vi "lab 9.vi"() -> ()   [LabVIEW 2021]
uses:
  <vilib>/MakerHub/LINX/Public/Peripherals/Analog/Analog Read 1 Chan.vi
  <vilib>/MakerHub/LINX/Public/Peripherals/Analog/Analog Read N Chans.vi
  <vilib>/MakerHub/LINX/Private/Local IO/LinxAnalogRead.vi
  <vilib>/MakerHub/LINX/Public/Utilities/Check Channel.vi
  <vilib>/MakerHub/LINX/Public/Utilities/Open Serial.vi
  <vilib>/MakerHub/LINX/Public/Sensors/Motion/Servo/Servo Set Pulse Width One Channel.vi
  <vilib>/MakerHub/LINX/Private/Utilties/Generate Error.vi
  <vilib>/MakerHub/LINX/LMH-LINX.lvlib
  <vilib>/MakerHub/LINX/Public/Sensors/Motion/Servo/Servo.lvlib
panel:
  in  "stop Button":bool
  in  "Servo Channel":u8
  in  "Analog Channel":u8
  out "Waveform Chart 2":dbl(graph)
  out "Waveform Chart":dbl(graph)
  in  "Serial Port":refnum<visa-resource-name>="N/A"
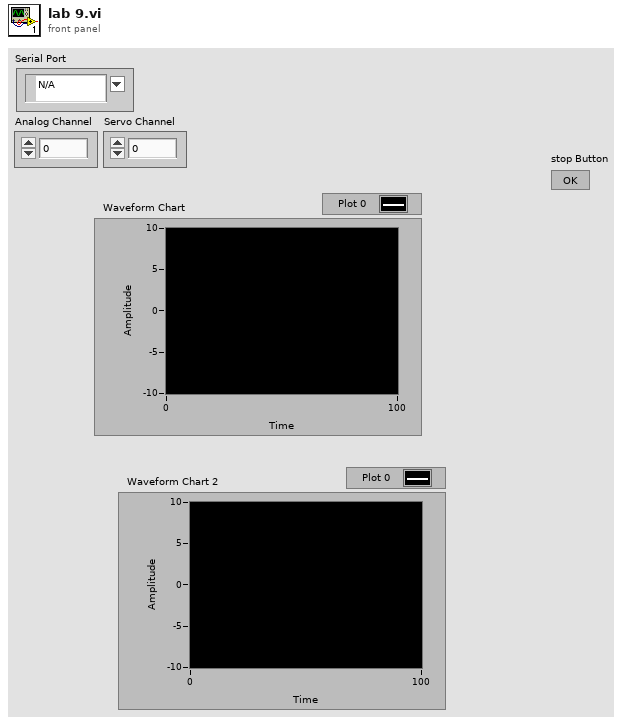
[diagram p1: front panel]
types:
  T1 = typedef "LMH-LINX.lvlib/LINX Ref.ctl" = cluster{"IO":T2, "Interface":T3, "LINX Device Config":T4}
  T2 = typedef "LMH-LINX.lvlib/Platform.ctl" = enum16{"Remote", "Local"}
  T3 = typedef "LMH-LINX.lvlib/Interface.ctl" = enum16{"Serial", "TCP"}
  T4 = typedef "LMH-LINX.lvlib/Device.lvlib/LINX Device Config.ctl" = cluster{"Interface":T3, "COM Port":refnum<visa-resource-name>, "TCP Configuration":T5, "Device Family":u8, "Device ID":u8, "Device Name":string, "TCP Ref":refnum<k5>, "Channels":T6}
  T5 = typedef "LMH-LINX.lvlib/Device.lvlib/TCP Config.ctl" = cluster{"IP Address":string, "Port":u16}
  T6 = typedef "LMH-LINX.lvlib/Channels.ctl" = cluster{"DI":u8[], "DO":u8[], "AI":u8[], "AO":u8[], "PWM":u8[], "QE":u8[], "UART":u8[], "I2C 2":u8[], "SPI":u8[], "CAN":u8[], "Servo":u8[], "AI Ref (V)":dbl, "AI Resolution (Bits)":u8, "AO Ref (V)":dbl, "AO Resolution (Bits)":u8}
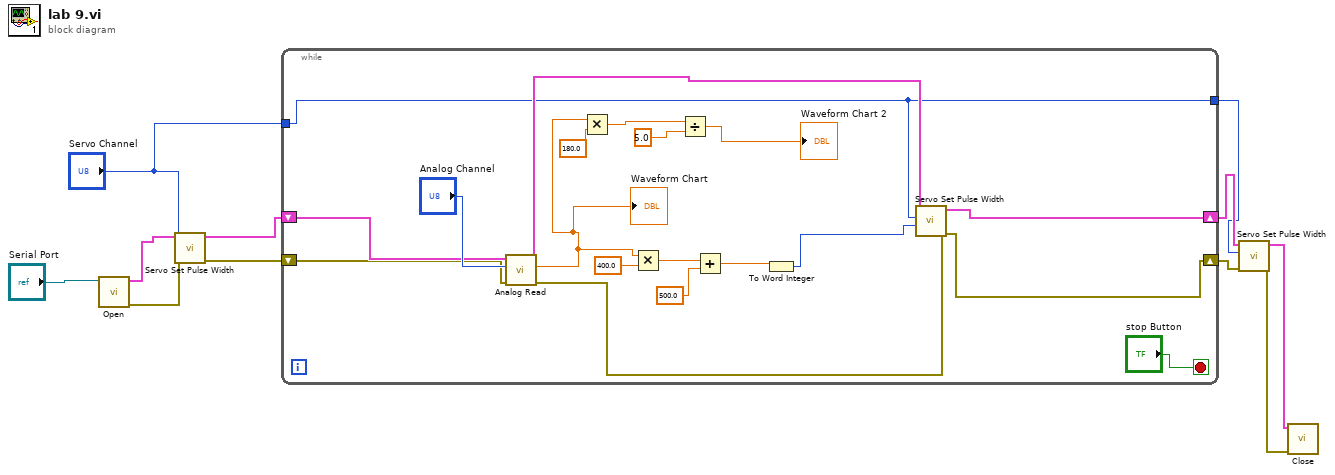
[diagram p0: block diagram]
diagram:
  n1 = call-poly <vilib>:"Open.vi"("Serial Port"="Serial Port") -> ("Error Out"=w8:errorcluster, "LINX Resource"=w10:T1)  [unwired: 8 in, 1 out]
  n2 = call-poly <vilib>:"Servo Set Pulse Width.vi"("Error In"=w8, "Servo Channel"="Servo Channel", "LINX Resource"=w10) -> ("Error Out"=w7:errorcluster, "LINX Resource"=w9:T1)  [unwired: 7 in]
  n3 = while {
    shift-right: [w26] -> w6
    shift-left: w9 -> [w29]
    shift-right: [w25] -> w3
    shift-left: w7 -> [w28]
    tunnel: "Servo Channel" -> [w14]
    tunnel: [w14] -> w1
    stop <- "stop Button" stop-if-true
    n4 = call-poly <vilib>:"Analog Read.vi"("Error In"=w28, "Analog Channel"="Analog Channel", "LINX Resource"=w29) -> ("Error Out"=w24:errorcluster, "Voltage"=w16:dbl, "LINX Resource"=w27:T1)  [unwired: 5 in, 1 out]
    "Waveform Chart" <- w16
    n5 = Multiply(x=w16, y=180.0) -> (x*y=w19:dbl)
    n6 = Multiply(x=w16, y=400.0) -> (x*y=w22:dbl)
    n7 = Divide(x=w19, y=5.0) -> (x/y=→"Waveform Chart 2":dbl)
    n8 = Add(x=w22, y=500.0) -> (x+y=w13:dbl)
    n9 = To Word Integer(number=w13) -> (16bit integer=w12:i16)
    n10 = call-poly <vilib>:"Servo Set Pulse Width.vi"("Error In"=w24, "Pulse Width (uS)"=w12, "Servo Channel"=w14, "LINX Resource"=w27) -> ("Error Out"=w25:errorcluster, "LINX Resource"=w26:T1)  [unwired: 6 in]
  }
  n11 = call-poly <vilib>:"Servo Set Pulse Width.vi"("Error In"=w3, "Servo Channel"=w1, "LINX Resource"=w6) -> ("Error Out"=w4:errorcluster, "LINX Resource"=w5:T1)  [unwired: 7 in]
  n12 = call <vilib>:"Close.vi"("Error In"=w4, "LINX Resource"=w5) -> ()  [unwired: 9 in, 1 out]
